vi "GoPro Poll Status.vi"(8 "error in (no error)":errorcluster, 11 "Gopro DevRef":T7) -> (0 "error out":errorcluster, 2 "GoPro Status":T1={"State"=enum."Menu", "Record Elapsed"="", "Record Remaining"=0, "On?"=FALSE, "sx"="", "cc"="", "cv"="", "se"="", "Recording?"=FALSE, "Video Files"=0, "Pics Remaining"=0, "Pic Files"=0, "FPS"=enum."120 FPS", "Resolution"=enum."1080p", "Spot Metering?"=FALSE, "Vid FOV"=enum."Wide", "Photo Resolution"=enum."10 MP W", "Beep Vol"=enum."OFF", "Battery Status"=0}, 3 "Output DevRef":T7)   [LabVIEW 2015]
uses:
  GoPro DevRef.ctl
  <vilib>/httpClient/ClientHandle.ctl
  GoPro Status.ctl
  GoPro Mode.ctl
  GoPro FPS.ctl
  GoPro Resolution.ctl
  GoPro Video FOV.ctl
  GoPro Photo Resolution.ctl
  <vilib>/httpClient/LabVIEWHTTPClient.lvlib
panel:
  out "sx":string
  out "cc":string
  out "cv":string
  out "se":string
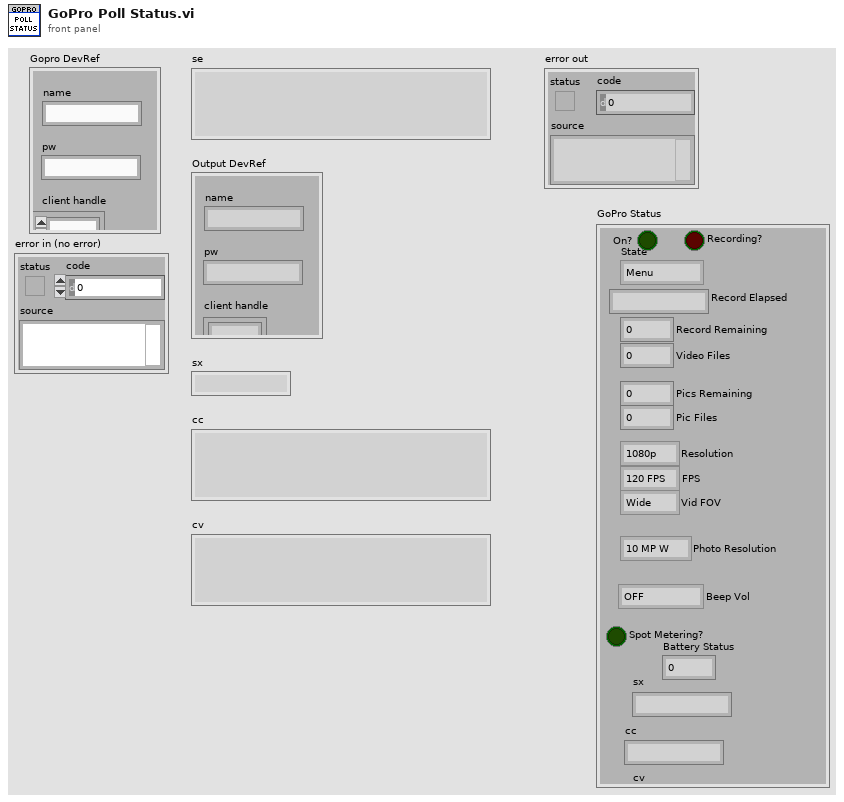
[diagram p1: front panel]
types:
  T1 = typedef "GoPro Status.ctl" = cluster{"State":T2, "Record Elapsed":string, "Record Remaining":i32, "On?":bool, "sx":string, "cc":string, "cv":string, "se":string, "Recording?":bool, "Video Files":i32, "Pics Remaining":i32, "Pic Files":i32, "FPS":T3, "Resolution":T4, "Spot Metering?":bool, "Vid FOV":T5, "Photo Resolution":T6, "Beep Vol":enum16{"OFF", "70%", "100%", "UNKOWN"}, "Battery Status":u8}
  T2 = typedef "GoPro Mode.ctl" = enum16{"UNKNOWN", "Video", "Photo", "Time Lapse", "Timer Delay", "Menu"}
  T3 = typedef "GoPro FPS.ctl" = enum16{"120 FPS", "60 FPS", "30 FPS", "UNKNOWN"}
  T4 = typedef "GoPro Resolution.ctl" = enum16{"1080p", "960p", "720p", "WVGA", "UNKNOWN"}
  T5 = typedef "GoPro Video FOV.ctl" = enum16{"Wide", "Medium", "Narrow", "UNKNOWN"}
  T6 = typedef "GoPro Photo Resolution.ctl" = enum16{"10 MP W", "7 MP W", "5 MP M", "UNKNOWN"}
  T7 = typedef "GoPro DevRef.ctl" = cluster{"name":string, "pw":string, "client handle":T8}
  T8 = typedef "LabVIEWHTTPClient.lvlib/ClientHandle.ctl" = refnum<k1>
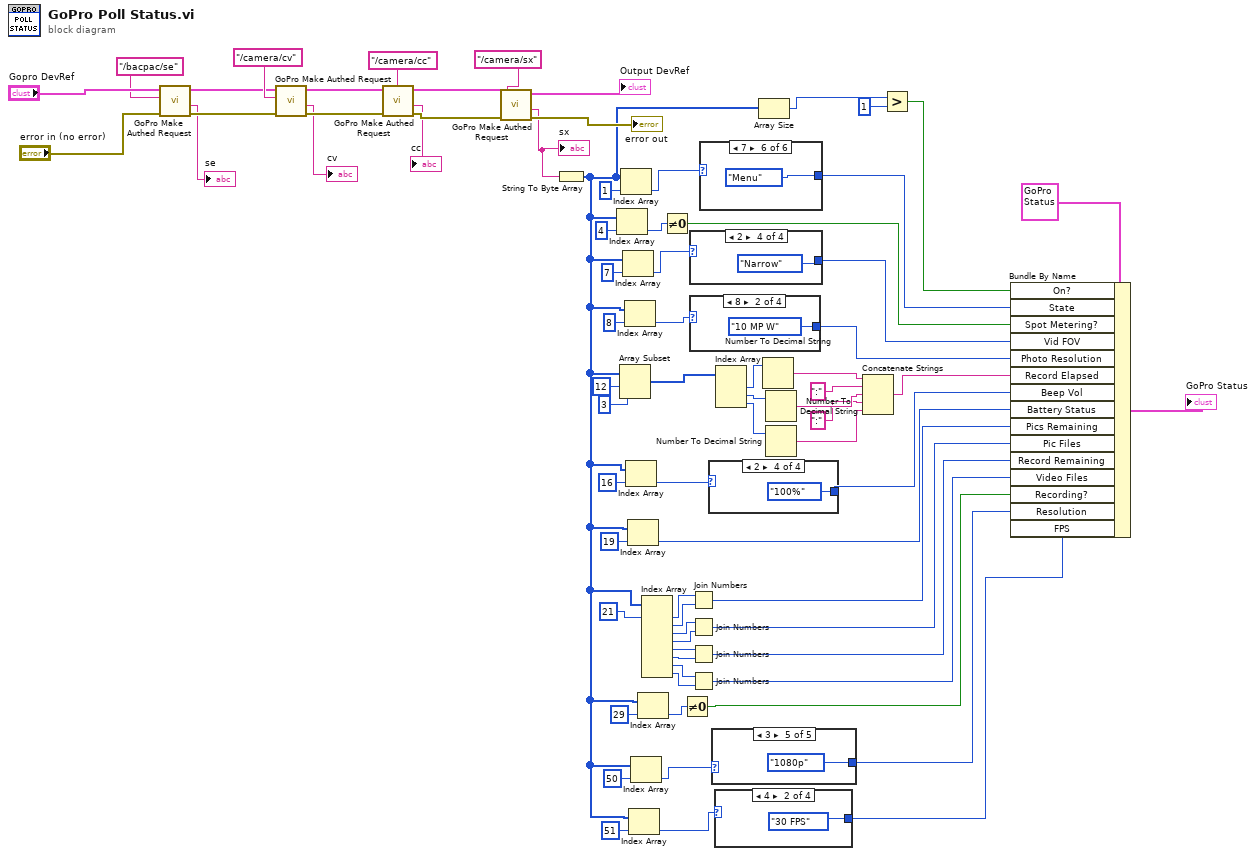
[diagram p0: block diagram]
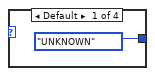
[diagram p2: hidden frame]
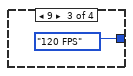
[diagram p3: hidden frame]
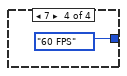
[diagram p4: hidden frame]
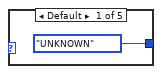
[diagram p5: hidden frame]
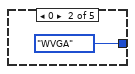
[diagram p6: hidden frame]
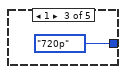
[diagram p7: hidden frame]
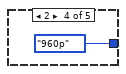
[diagram p8: hidden frame]
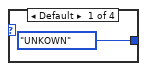
[diagram p9: hidden frame]
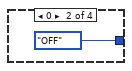
[diagram p10: hidden frame]
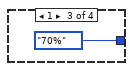
[diagram p11: hidden frame]
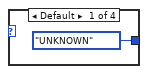
[diagram p12: hidden frame]
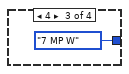
[diagram p13: hidden frame]
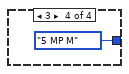
[diagram p14: hidden frame]
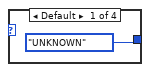
[diagram p15: hidden frame]
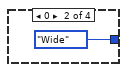
[diagram p16: hidden frame]
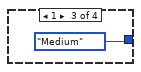
[diagram p17: hidden frame]
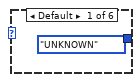
[diagram p18: hidden frame]
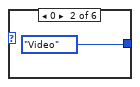
[diagram p19: hidden frame]
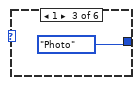
[diagram p20: hidden frame]
diagram:
  n1 = call "GoPro Make Authed Request.vi"("error in (no error)"="error in (no error)", "url"="/bacpac/se", "Gopro DevRef"="Gopro DevRef") -> ("error out"=w65:errorcluster, "body"=→"se":string, "Output DevRef"=w68:T7)  [unwired: 5 in, 1 out]
  n2 = call "GoPro Make Authed Request.vi"("error in (no error)"=w65, "url"="/camera/cv", "Gopro DevRef"=w68) -> ("error out"=w64:errorcluster, "body"=→"cv":string, "Output DevRef"=w69:T7)  [unwired: 5 in, 1 out]
  n3 = call "GoPro Make Authed Request.vi"("error in (no error)"=w64, "url"="/camera/cc", "Gopro DevRef"=w69) -> ("error out"=w63:errorcluster, "body"=→"cc":string, "Output DevRef"=w70:T7)  [unwired: 5 in, 1 out]
  n4 = call "GoPro Make Authed Request.vi"("error in (no error)"=w63, "url"="/camera/sx", "Gopro DevRef"=w70) -> ("error out"=→"error out":errorcluster, "body"=w43:string, "Output DevRef"=→"Output DevRef":T7)  [unwired: 5 in, 1 out]
  "sx" <- w43
  n5 = String To Byte Array(string=w43) -> (unsigned byte array=w2:u8[])
  n6 = Index Array(array=w2, index=4) -> (element=w38:u8)
  n7 = Array Subset(array=w2, index=12, length=3) -> (w57:u8[])
  n8 = Index Array(array=w2, index=1) -> (element=w58:u8)
  n9 = Index Array(array=w2, index=7) -> (element=w34:u8)
  n10 = Index Array(array=w2, index=8) -> (element=w31:u8)
  n11 = Index Array(array=w2, index=16) -> (element=w28:u8)
  n12 = Index Array(array=w2, index=19) -> (element=w1:u8)
  n13 = Index Array(array=w2, index=51) -> (element=w6:u8)
  n14 = Index Array(array=w2, index=50) -> (element=w9:u8)
  n15 = Index Array(array=w2, index=29) -> (element=w12:u8)
  n16 = Index Array(array=w2, index #1=21 ("index")) -> (element #1=w25:u8, element #2=w26:u8, element #3=w22:u8, element #4=w21:u8, element #5=w19:u8, element #6=w18:u8, element #7=w16:u8, element #8=w15:u8)  [unwired: 7 in]
  n17 = Not Equal To 0?(x=w38) -> (x != 0?=w36:bool)
  n18 = Not Equal To 0?(x=w12) -> (x != 0?=w11:bool)
  n19 = Join Numbers(hi=w25, lo=w26) -> ((hi.lo)=w23:u16)
  n20 = Join Numbers(hi=w22, lo=w21) -> ((hi.lo)=w20:u16)
  n21 = Join Numbers(hi=w19, lo=w18) -> ((hi.lo)=w17:u16)
  n22 = Join Numbers(hi=w16, lo=w15) -> ((hi.lo)=w14:u16)
  n23 = case shown="2" w34 {
    tunnel: [GoPro_Video_FOV."UNKNOWN" ("Vid FOV") GoPro_Video_FOV."Wide" ("Vid FOV") GoPro_Video_FOV."Medium" ("Vid FOV") GoPro_Video_FOV."Narrow" ("Vid FOV")] -> w33
    frame Default {
    }
    frame 0 {
    }
    frame 1 {
    }
    frame 2 {
    }
  }
  n24 = case shown="8" w31 {
    tunnel: [GoPro_Photo_Resolution."UNKNOWN" ("Photo Resolution") GoPro_Photo_Resolution."10 MP W" ("Photo Resolution") GoPro_Photo_Resolution."7 MP W" ("Photo Resolution") GoPro_Photo_Resolution."5 MP M" ("Photo Resolution")] -> w30
    frame Default {
    }
    frame 8 {
    }
    frame 4 {
    }
    frame 3 {
    }
  }
  n25 = case shown="7" w58 {
    tunnel: [GoPro_Mode."UNKNOWN" GoPro_Mode."Video" GoPro_Mode."Photo" GoPro_Mode."Time Lapse" GoPro_Mode."Timer Delay" GoPro_Mode."Menu"] -> w37
    frame Default {
    }
    frame 0 {
    }
    frame 1 {
    }
    frame 2 {
    }
    frame 3 {
    }
    frame 7 {
    }
  }
  n26 = case shown="2" w28 {
    tunnel: [enum16{"OFF", "70%", "100%", "UNKOWN"}."UNKOWN" ("Beep Vol") enum16{"OFF", "70%", "100%", "UNKOWN"}."OFF" ("Beep Vol") enum16{"OFF", "70%", "100%", "UNKOWN"}."70%" ("Beep Vol") enum16{"OFF", "70%", "100%", "UNKOWN"}."100%" ("Beep Vol")] -> w27
    frame Default {
    }
    frame 0 {
    }
    frame 1 {
    }
    frame 2 {
    }
  }
  n27 = case shown="3" w9 {
    tunnel: [GoPro_Resolution."UNKNOWN" ("Resolution") GoPro_Resolution."WVGA" ("Resolution") GoPro_Resolution."720p" ("Resolution") GoPro_Resolution."960p" ("Resolution") GoPro_Resolution."1080p" ("Resolution")] -> w8
    frame Default {
    }
    frame 0 {
    }
    frame 1 {
    }
    frame 2 {
    }
    frame 3 {
    }
  }
  n28 = case shown="4" w6 {
    tunnel: [GoPro_FPS."UNKNOWN" ("FPS") GoPro_FPS."30 FPS" ("FPS") GoPro_FPS."120 FPS" ("FPS") GoPro_FPS."60 FPS" ("FPS")] -> w5
    frame Default {
    }
    frame 4 {
    }
    frame 9 {
    }
    frame 7 {
    }
  }
  n29 = Index Array(array=w57) -> (element #1=w56:u8, element #2=w55:u8, element #3=w54:u8)  [unwired: 3 in]
  n30 = Array Size(array=w2) -> (size(s)=w46:i32)
  n31 = Number To Decimal String(number=w56) -> (decimal integer string=w53:string)  [unwired: 1 in]
  n32 = Number To Decimal String(number=w55) -> (decimal integer string=w51:string)  [unwired: 1 in]
  n33 = Number To Decimal String(number=w54) -> (decimal integer string=w49:string)  [unwired: 1 in]
  n34 = Concatenate Strings(w53, ":", w51, ":", w49) -> (w47:string)
  n35 = Greater?(x=w46, y=1) -> (0:w44:bool)
  n36 = Bundle By Name(cluster=T1 {"State"=enum."Menu", "Record Elapsed"="", "Record Remaining"=0, "On?"=FALSE, "sx"="", "cc"="", "cv"="", "se"="", "Recording?"=FALSE, "Video Files"=0, "Pics Remaining"=0, "Pic Files"=0, "FPS"=enum."120 FPS", "Resolution"=enum."1080p", "Spot Metering?"=FALSE, "Vid FOV"=enum."Wide", "Photo Resolution"=enum."10 MP W", "Beep Vol"=enum."OFF", "Battery Status"=0} ("GoPro Status"), "On?"=w44, "State"=w37, "Spot Metering?"=w36, "Vid FOV"=w33, "Photo Resolution"=w30, "Record Elapsed"=w47, "Beep Vol"=w27, "Battery Status"=w1, "Pics Remaining"=w23, "Pic Files"=w20, "Record Remaining"=w17, "Video Files"=w14, "Recording?"=w11, "Resolution"=w8, "FPS"=w5) -> (→"GoPro Status":T1)
